vi "Setup Example Mono.vi"(8 "error in (no error)":errorcluster, 11 "Mono In":refnum<class "Monochromator.lvclass">) -> (0 "error out":errorcluster, 1 "device is open?":bool, 2 "Module Was Already Running?":bool, 3 "Mono Out":refnum<class "Monochromator.lvclass">)   [LabVIEW 2020, in "Examples.lvlib"]
doc: "Setup for the mono examples."
uses:
  Examples.lvlib
  Classes/DeviceManager/DeviceManager.lvlib
  Classes/Mono/Monochromator.lvclass
panel:
  # "Connector Pane"
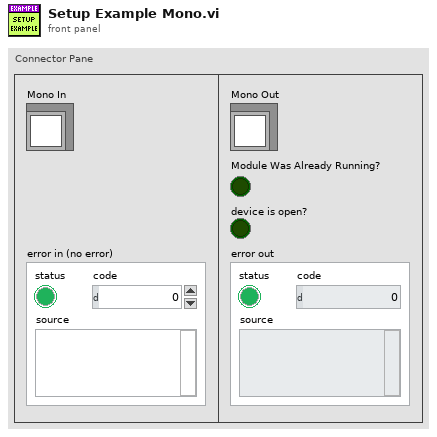
[diagram p1: front panel]
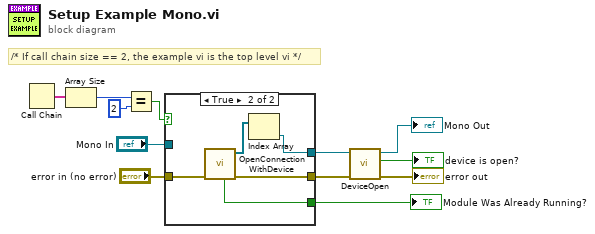
[diagram p0: block diagram]
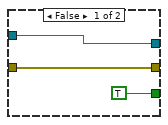
[diagram p2: hidden frame]
diagram:
  # "/* If call chain size == 2, the example vi is the top level vi */"
  n1 = Call Chain() -> (call chain=w9:string[])
  n2 = Array Size(array=w9) -> (size(s)=w10:i32)
  n3 = Equal?(x=w10, y=2) -> (x = y?=w12:bool)
  n4 = case shown="True" w12 {
    tunnel: [w15 w19] -> w5
    tunnel: "Mono In" -> [w15 _]
    tunnel: [TRUE ("Module Was Already Running?") w20] -> w8
    tunnel: "error in (no error)" -> [w14 w18]
    tunnel: [w14 w17] -> w4
    frame False {
    }
    frame True {
      n5 = call "OpenConnectionWithDevice.vi"("error in"=w18) -> ("error out"=w17:errorcluster, "Monos"=w16:refnum<class "Monochromator.lvclass">[], "Module Was Already Running?"=w20:bool)  [unwired: 6 in, 2 out]
      n6 = Index Array(array=w16) -> (element=w19:refnum<class "Monochromator.lvclass">)  [unwired: 1 in]
    }
  }
  "Module Was Already Running?" <- w8
  n7 = call-dynamic "DeviceOpen.vi"("error in (no error)"=w4, "Monochromator in"=w5) -> ("error out"=→"error out":errorcluster, "device is open?"=→"device is open?":bool, "Monochromator out"=→"Mono Out":refnum<class "Monochromator.lvclass">)  [unwired: 6 in, 1 out]
